vi "TestFiltering.vi"() -> ()   [LabVIEW 2011]
uses:
  <vilib>/userdefined/High Color/nirio_resource_hc.ctl
  <vilib>/LabVIEW Targets/FPGA/RIO/nirio_PxiTriggers.ctl
  <vilib>/FPGAPlugInAG/PXIe-7965R/niLvFpga_Open_PXIe-7965R.vi
  <vilib>/FPGAPlugInAG/PXIe-7965R/niLvFpga_Reset_PXIe-7965R.vi
  <vilib>/FPGAPlugInAG/PXIe-7965R/niLvFpga_Run_PXIe-7965R.vi
  <vilib>/LabVIEW Targets/FPGA/RIO/nirioReserveTrigger.vi
  <vilib>/LabVIEW Targets/FPGA/79XXR/Private/79XXR_Method_IOModuleStatusImpl.vi
  <vilib>/Utility/error.llb/Error Cluster From Error Code.vi
  <vilib>/rvi/errors/niLvFpgaAdjustHostInterfaceError.vi
  <vilib>/express/express analysis/Spectral/Block/exnSpectralBlock spectral measurements PSD poly.vi
  <vilib>/express/express analysis/Spectral/Block/exnSpectralBlock spectral measurements PSD WFM.vi
  <vilib>/rvi/interface/nirviOpenFPGA/nirviOpenFPGA.xnode
  FPGA Bitfiles/Acquisition_FPGATarget_FilteringTest_B0B7068A.lvbitx
  <vilib>/rvi/interface/nirviMethod/nirviMethod.xnode
  <vilib>/FPGA/interface/niFpgaViExecutionMode.ctl
  <vilib>/express/express analysis/Spectral/XNode/ExpressSpectralMeasurementsBlockNode.xnode
  <vilib>/rvi/interface/nirviReadWriteControl/nirviReadWriteControl.xnode
  <vilib>/rvi/errors/niLvFpgaMergeErrorWithErrorCode.vi
  <vilib>/FPGAPlugInAG/PXIe-7965R/niLvFpga_ConfigureFifo_PXIe-7965R.vi
  <vilib>/FPGAPlugInAG/PXIe-7965R/niLvFpga_StartFifo_PXIe-7965R.vi
  <vilib>/FPGAPlugInAG/PXIe-7965R/niLvFpga_ReadFifo_PXIe-7965R.vi
  NiFpgaLv.dll
panel:
  in  "Offset":i32=800
  out "LoopTickTime":u32
  in  "Filter":bool
  out "Waveform Graph":cluster{"f0":dbl, "df":dbl, "magnitude":dbl[]}(graph)
  out "FFT - (RMS)":cluster{"f0":dbl, "df":dbl, "magnitude":dbl[]}
  out "S/s":dbl
  out "Waveform Chart":i32[](graph)
  out "Timed Out?":bool
  in  "stop":bool
  out "Data":i16[](array[numeric])
  out "error out":errorcluster
  in  "error in (no error)":errorcluster
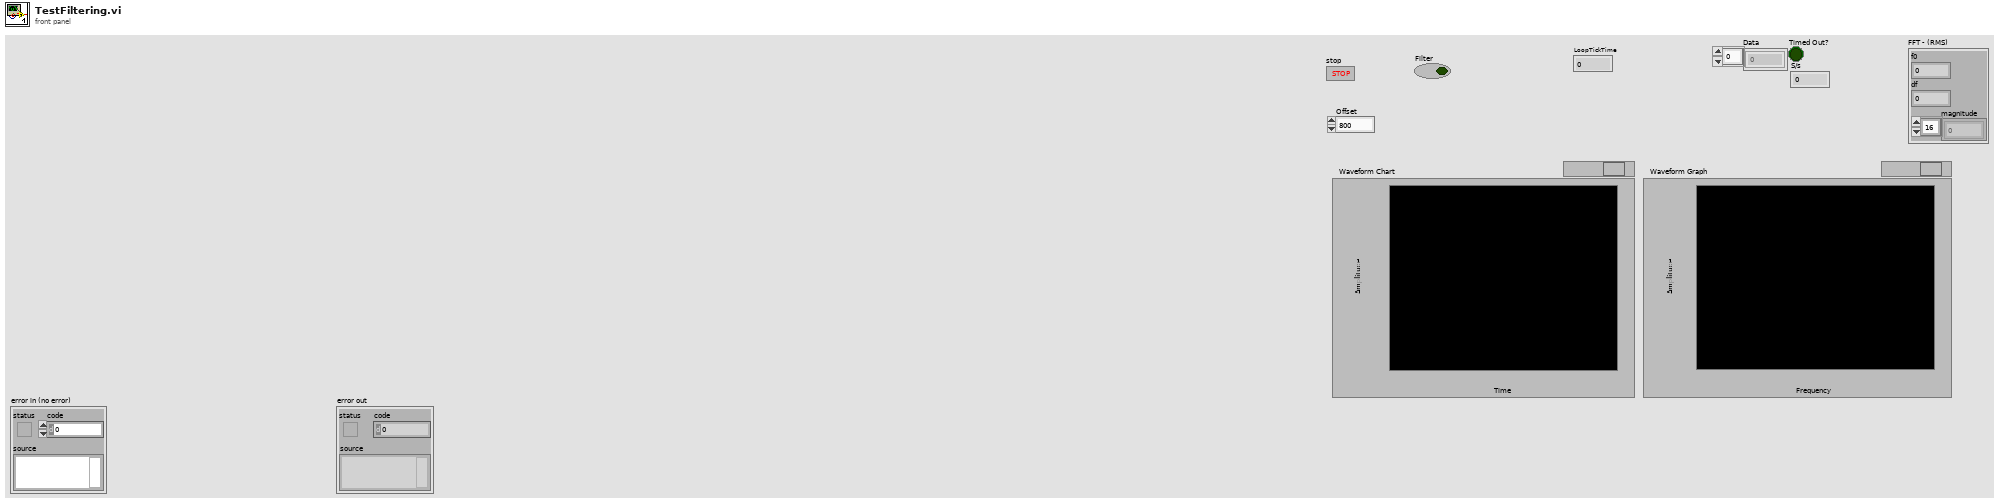
[diagram p1: front panel]
types:
  T1 = typedef "nirio_resource_hc.ctl" = tag
  T2 = typedef "niFpgaViExecutionMode.ctl" = enum16{"FPGA Target", "Development Computer with Simulated I/O", "Development Computer with Real I/O", "Third-Party Simulator"}
  T3 = typedef "nirio_PxiTriggers.ctl" = u16
  T4 = cluster{"averaging mode":u16, "weighting mode":u16, "number of averages":u32}
  T5 = cluster{"dB On (F)":bool, "unwrap phase (F)":bool, "convert to degree (F)":bool}
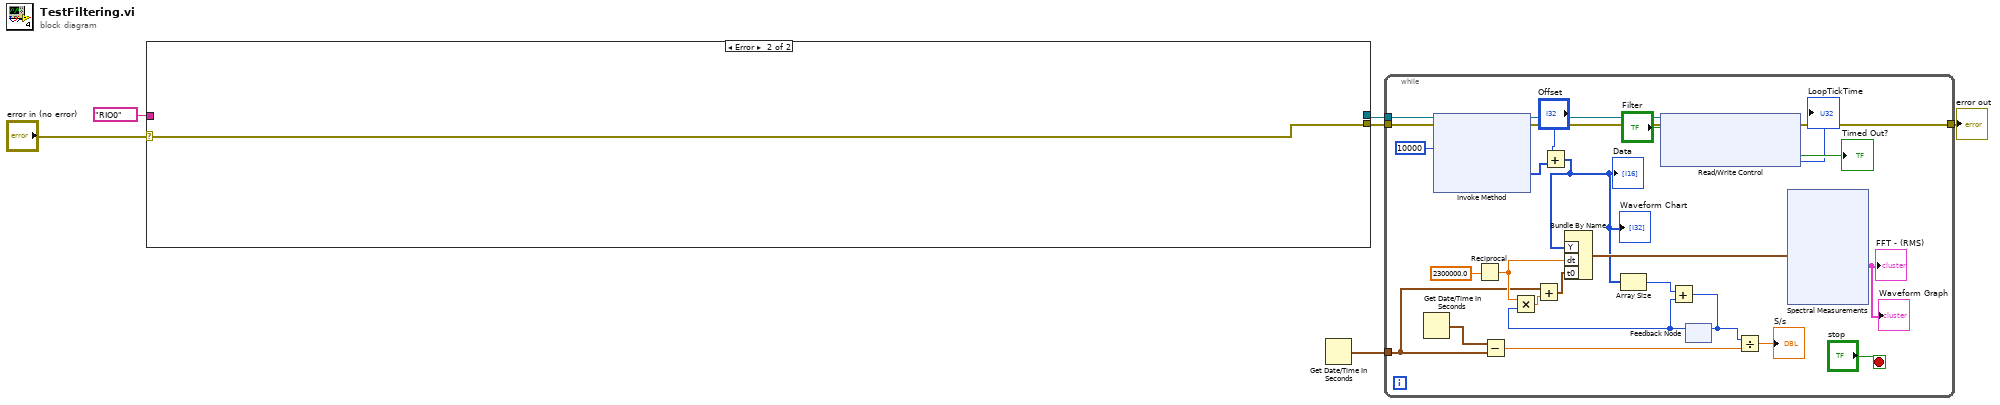
[diagram p0: block diagram]
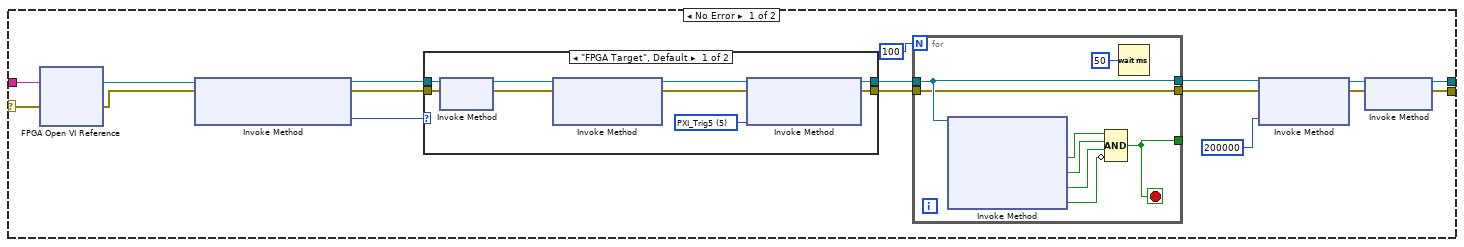
[diagram p2: hidden frame]
diagram:
  n1 = case shown="Error" "error in (no error)" {
    selector: "error in (no error)" -> [w21 w43]
    tunnel: [w9 w43] -> w3
    tunnel: T1 "RIO0" ("RIO Device") -> [w19 _]
    tunnel: [w7 _] -> w4
    frame No Error {
      n2 = xnode "FPGA Open VI Reference"("error in"=w21, "resource name"=w19) -> ("FPGA VI Reference Out"=w18:refnum<k20>, "error out"=w8:errorcluster)
      n3 = xnode "Invoke Method"("FPGA VI Reference In"=w18, "error in"=w8) -> ("FPGA VI Reference Out"=w23:refnum<k20>, "error out"=w20:errorcluster, "FPGA VI Execution Mode"=w22:T2)
      n4 = case shown="\"FPGA Target\", Default" w22 {
        tunnel: [w36 w42] -> w17
        tunnel: w23 -> [w40 w42]
        tunnel: w20 -> [w35 w41]
        tunnel: [w32 w41] -> w16
        frame "FPGA Target", Default {
          w38 = T3 5 items=["PXI_Trig0", "PXI_Trig1", "PXI_Trig2", "PXI_Trig3", "PXI_Trig4", "PXI_Trig5", "PXI_Trig6", "PXI_Trig7"] ("Trigger")
          n5 = xnode "Invoke Method"("FPGA VI Reference In"=w40, "error in"=w35) -> ("FPGA VI Reference Out"=w39:refnum<k20>, "error out"=w34:errorcluster)
          n6 = xnode "Invoke Method"("FPGA VI Reference In"=w39, "error in"=w34) -> ("FPGA VI Reference Out"=w37:refnum<k20>, "error out"=w33:errorcluster)  [unwired: 1 in]
          n7 = xnode "Invoke Method"("FPGA VI Reference In"=w37, "error in"=w33, "Trigger"=w38) -> ("FPGA VI Reference Out"=w36:refnum<k20>, "error out"=w32:errorcluster)
        }
        frame "Development Computer with Simulated I/O" {
        }
      }
      n8 = for {
        N: 100 -> [_]
        tunnel: w17 -> [w25]
        tunnel: w16 -> [w24]
        tunnel: [w26] -> _
        tunnel: [w25] -> w13
        tunnel: [w24] -> w12
        stop <- w26 stop-if-true
        n9 = xnode "Invoke Method"("FPGA VI Reference In"=w25) -> ("IO Module Present?"=w31:bool, "Power Enabled?"=w30:bool, "IO Enabled?"=w29:bool, "IO Module Mismatch?"=w28:bool)  [unwired: 1 in, 2 out]
        n10 = Compound Arithmetic op=AND(w31, w30, w29, invert w28) -> (w26:bool)
        n11 = Wait (ms)(milliseconds to wait=u32 50) -> ()  [unwired: 1 out]
      }
      n12 = xnode "Invoke Method"("FPGA VI Reference In"=w13, "error in"=w12, "Depth"=u32 200000) -> ("FPGA VI Reference Out"=w11:refnum<k20>, "error out"=w10:errorcluster)
      n13 = xnode "Invoke Method"("FPGA VI Reference In"=w11, "error in"=w10) -> ("FPGA VI Reference Out"=w7:refnum<k20>, "error out"=w9:errorcluster)
    }
    frame Error {
    }
  }
  n14 = Get Date/Time In Seconds() -> (seconds since 1Jan1904=w1:timestamp)
  n15 = while {
    tunnel: w4 -> [w69]
    tunnel: w3 -> [w68]
    tunnel: [w63] -> w2
    tunnel: w1 -> [w51]
    stop <- "stop" stop-if-true
    n16 = Get Date/Time In Seconds() -> (seconds since 1Jan1904=w57:timestamp)
    n17 = xnode "Invoke Method"("FPGA VI Reference In"=w69, "error in"=w68, "Number of Elements"=u32 10000) -> ("FPGA VI Reference Out"=w65:refnum<k20>, "error out"=w64:errorcluster, "Data"=w48:i16[])  [unwired: 1 in, 1 out]
    n18 = Reciprocal(x=2300000.0) -> (1/x=w54:dbl)
    n19 = Subtract(x=w57, y=w51) -> (x-y=w56:dbl)
    n20 = Add(x="Offset", y=w48) -> (x+y=w46:i32[])
    "Data" <- w46
    "Waveform Chart" <- w46
    n21 = Array Size(array=w46) -> (size(s)=w61:i32)
    n22 = xnode "Read/Write Control"("FPGA VI Reference In"=w65, "error in"=w64, "Filter"="Filter") -> ("error out"=w63:errorcluster, "Timed Out?"=→"Timed Out?":bool, "LoopTickTime"=→"LoopTickTime":u32)  [unwired: 1 out]
    n23 = feedback #1() -> (w53:i32)  [unwired: 1 in]
    n24 = Multiply(x=w54, y=w53) -> (x*y=w52:dbl)
    n25 = Add(x=w51, y=w52) -> (x+y=w50:timestamp)
    n26 = Bundle By Name("Y"=w46, "dt"=w54, "t0"=w50) -> (w49:waveform(i32))  [unwired: 1 in]
    n27 = Add(x=w61, y=w53) -> (x+y=w60:i32)
    n28 = feedback-in #1(w60) -> ()
    n29 = Divide(x=w60, y=w56) -> (x/y=→"S/s":dbl)
    n30 = xnode "Spectral Measurements"("Signals"=w49) -> ("PSD"=→"FFT - (RMS)" →"Waveform Graph":cluster{"f0":dbl, "df":dbl, "magnitude":dbl[]})  [unwired: 2 in, 2 out]
  }
  "error out" <- w2
